vi "SetTransparency(U8).vi"(8 "error in":errorcluster, 9 "Run VI Transparently (T)":bool=TRUE, 10 "Transparency (%)":u8, 11 "VI Reference (calling VI)":refnum<vi>) -> (0 "error out":errorcluster, 3 "dup VI Reference":refnum<vi>)   [LabVIEW 2012]
doc: "Sets the transparency value (in %) of the VI from which a reference has been provided.\n\nVariant (%) can be a numeric or a string containing a number. This allows the use of string-based arguments without the need to convert to a number.\n\nFront panel transparency of 0% means opaque, while 100% is completely transparent."
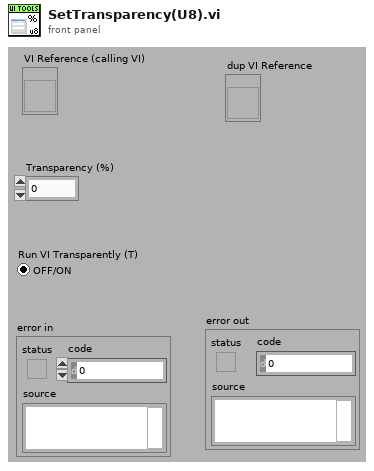
[diagram p1: front panel]
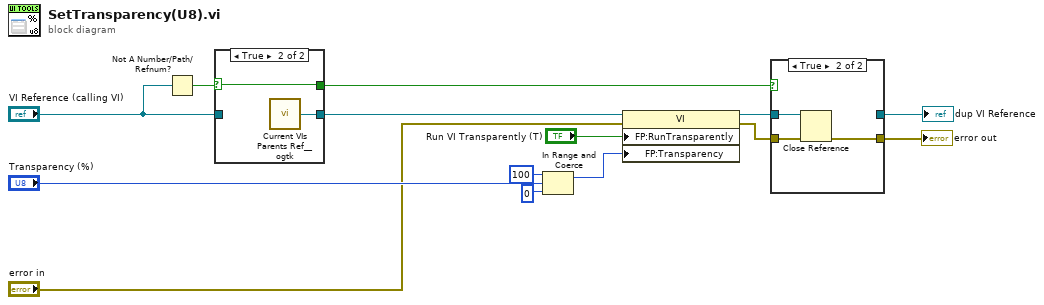
[diagram p0: block diagram]
diagram:
  n1 = Not A Number/Path/Refnum?(number/path/refnum="VI Reference (calling VI)") -> (NaN/Path/Refnum?=w14:bool)
  n2 = case shown="True" w14 {
    selector: w14 -> [w15 w17]
    tunnel: "VI Reference (calling VI)" -> [w16 _]
    tunnel: [w16 w18] -> w10
    tunnel: [w15 w17] -> w2
    frame False {
    }
    frame True {
      n3 = call <userlib>:"Current VIs Parents Ref__ogtk.vi"() -> ("Calling VI's Reference"=w18:refnum<vi>)  [unwired: 2 out]
    }
  }
  n4 = In Range and Coerce(upper limit=u8 100 ("Front Panel Window:Transparency"), x="Transparency (%)", lower limit=u8 0 ("Front Panel Window:Transparency")) -> (coerced(x)=w9:u8)  [unwired: 1 out]
  n5 = property class="VI"(reference=w10, error in="error in", "FP:RunTransparently"="Run VI Transparently (T)", "FP:Transparency"=w9) -> (reference out=w6:refnum<vi>, error out=w5:errorcluster)
  n6 = case shown="True" w2 {
    tunnel: w6 -> [w20 w23]
    tunnel: [w20 _] -> w3
    tunnel: w5 -> [w19 w22]
    tunnel: [w19 w21] -> w4
    frame False {
    }
    frame True {
      n7 = Close Reference(reference=w23, error in (no error)=w22) -> (error out=w21:errorcluster)
    }
  }
  "dup VI Reference" <- w3
  "error out" <- w4
